vi "1-4.vi"() -> ()   [LabVIEW 2018]
panel:
  out "LED3":bool
  out "LED2":bool
  out "LED1":bool
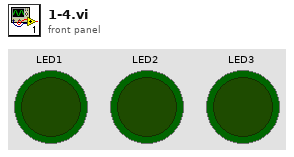
[diagram p1: front panel]
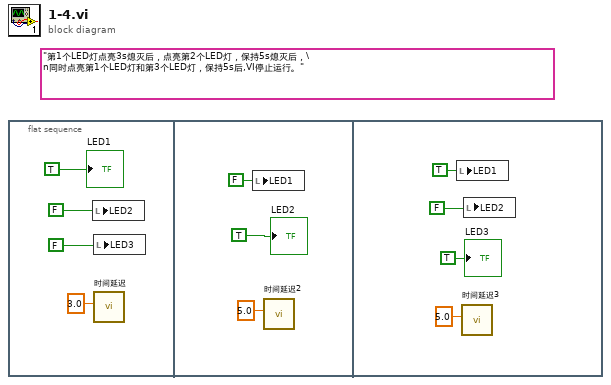
[diagram p0: block diagram]
diagram:
  (unwired) "第1个LED灯点亮3s熄灭后，点亮第2个LED灯，保持5s熄灭后，\n同时点亮第1个LED灯和第3个LED灯，保持5s后,VI停止运行。"
  n1 = flat-sequence {
    frame #0 {
      n2 = local write "LED2"(FALSE) -> ()
      n3 = local write "LED3"(FALSE) -> ()
      n4 = call "时间延迟"("Delay Time (s)"=3.0) -> ()  [unwired: 10 in, 1 out]
      "LED1" <- TRUE
    }
    frame #1 {
      n5 = local write "LED1"(FALSE ("LED1")) -> ()
      n6 = call "时间延迟2"("Delay Time (s)"=5.0) -> ()  [unwired: 10 in, 1 out]
      "LED2" <- TRUE ("LED1 2")
    }
    frame #2 {
      n7 = local write "LED1"(TRUE ("LED1")) -> ()
      n8 = call "时间延迟3"("Delay Time (s)"=5.0) -> ()  [unwired: 10 in, 1 out]
      n9 = local write "LED2"(FALSE) -> ()
      "LED3" <- TRUE ("LED1 3")
    }
  }
